vi "esp_web_server_get.vi"() -> (0 "error out":errorcluster, 1 "Data":string[](array[string]), 2 "Cleaned Content":string, 3 "HTML Content":string)   [LabVIEW 2017]
uses:
  <vilib>/httpClient/LabVIEWHTTPClient.lvlib
panel:
  out "Waiting for Message":bool
  in  "error in (no error)":errorcluster
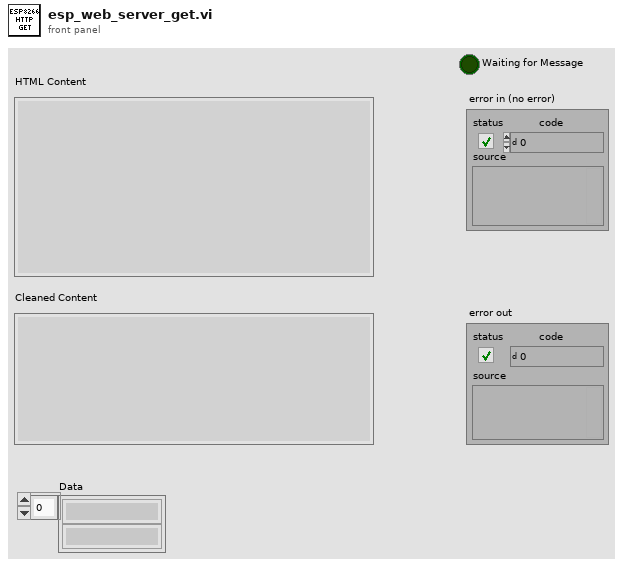
[diagram p1: front panel]
types:
  T1 = typedef "LabVIEWHTTPClient.lvlib/ClientHandle.ctl" = refnum<k1>
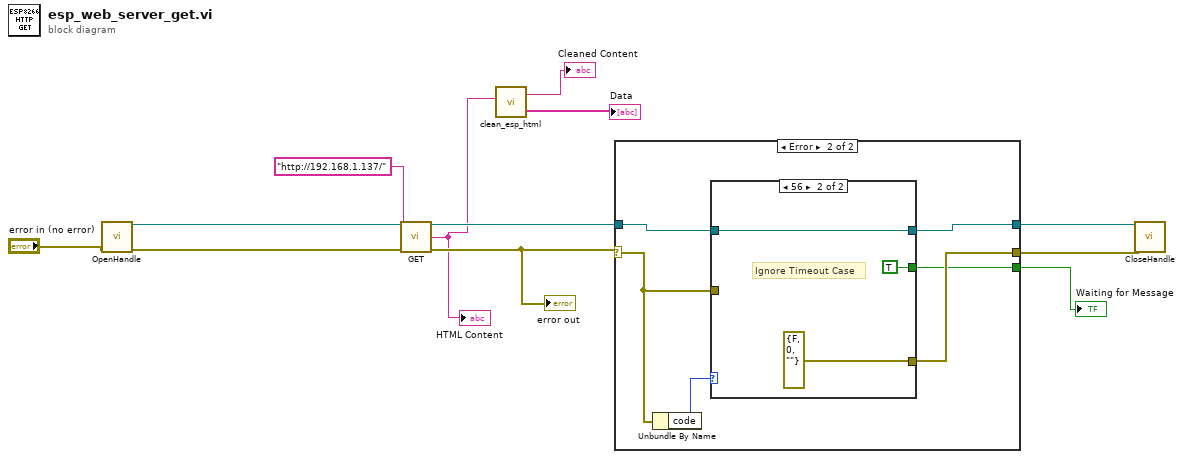
[diagram p0: block diagram]
diagram:
  n1 = call <vilib>:"OpenHandle.vi"("error in (no error)"="error in (no error)") -> ("client handle out"=w12:T1, "error out"=w11:errorcluster)  [unwired: 13 in]
  n2 = call <vilib>:"GET.vi"("client handle"=w12, "url"="http://192.168.1.137/", "error in (no error)"=w11) -> ("client handle out"=w8:T1, "body"=w3:string, "error out"=w4:errorcluster)  [unwired: 9 in, 1 out]
  "HTML Content" <- w3
  "error out" <- w4
  n3 = call "clean_esp_html.vi"("Body"=w3) -> ("Cleaned Body"=→"Cleaned Content":string, "appended array"=→"Data":string[])
  n4 = case shown="Error" w4 {
    selector: w4 -> [w13 w19]
    tunnel: w8 -> [w14 w18]
    tunnel: [w14 w17] -> w7
    tunnel: [w13 w16] -> w6
    tunnel: [_ w15] -> w5
    frame No Error {
    }
    frame Error {
      n5 = Unbundle By Name(w19) -> ("code"=w20:i32)
      n6 = case shown="56" w20 {
        tunnel: [w21 errorcluster {"status"=FALSE, "code"=0, "source"=""} ("error constant")] -> w16
        tunnel: w19 -> [w21 _]
        tunnel: [w22 w24] -> w17
        tunnel: w18 -> [w22 w24]
        tunnel: [_ TRUE ("Waiting for Message")] -> w15
        frame Default {
        }
        frame 56 {
          # "Ignore Timeout Case"
        }
      }
    }
  }
  "Waiting for Message" <- w5
  n7 = call <vilib>:"CloseHandle.vi"("client handle"=w7, "error in (no error)"=w6) -> ()  [unwired: 13 in, 1 out]
